vi "Test - FGV - Test Results.vi"(7 "Get/Set":T2, 8 "error in (no error)":errorcluster, 10 "Step Result":T1={"Step Name"="", "Value"=0.0, "Success ?"=TRUE, "Stop Seq ?"=FALSE, "Abort"=FALSE, "Sr.No"=0}) -> (0 "error out":errorcluster, 2 "Results":T1[](array[typedef]))   [LabVIEW 2017]
uses:
  Test - Step Result.ctl
  Controls/RT- Get Set.ctl
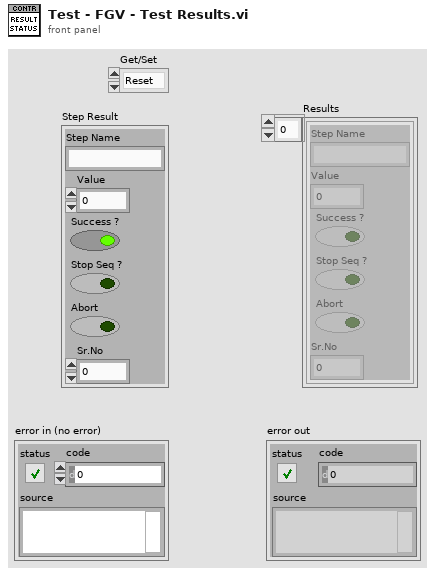
[diagram p1: front panel]
types:
  T1 = typedef "Test - Step Result.ctl" = cluster{"Step Name":string, "Value":dbl, "Success ?":bool, "Stop Seq ?":bool, "Abort":bool, "Sr.No":i32}
  T2 = typedef "RT- Get Set.ctl" = enum16{"Reset", "Get", "Set"}
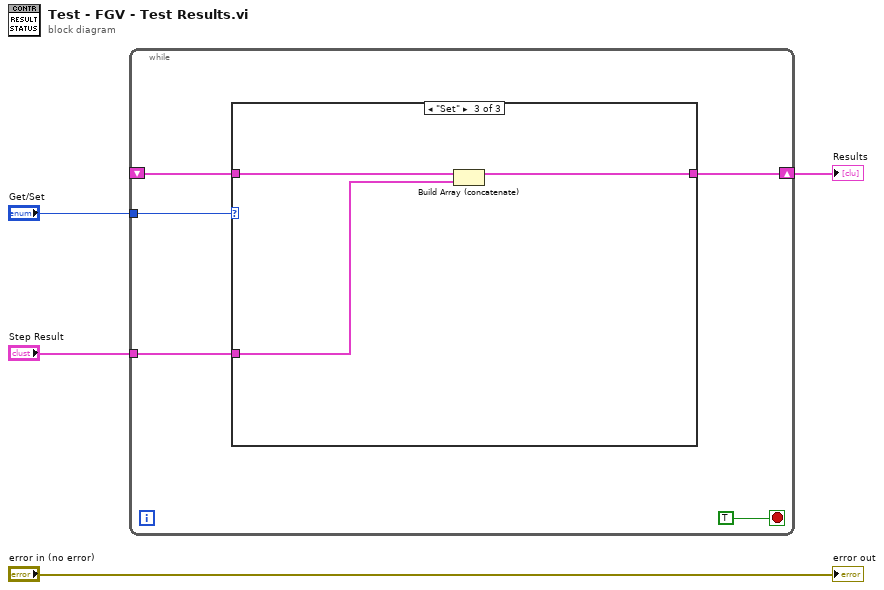
[diagram p0: block diagram]
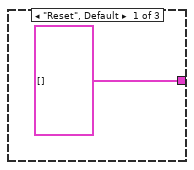
[diagram p2: hidden frame]
diagram:
  n1 = while {
    tunnel: "Get/Set" -> [w8]
    shift-right: [w7] -> w1
    shift-left: _ -> [w6]
    tunnel: "Step Result" -> [w5]
    stop <- TRUE stop-if-true
    n2 = case shown="\"Set\"" w8 {
      tunnel: [T1[] [] w11 w12] -> w7
      tunnel: w6 -> [_ w11 w14]
      tunnel: w5 -> [_ _ w13]
      frame "Reset", Default {
      }
      frame "Get" {
      }
      frame "Set" {
        n3 = Build Array (concatenate)(w14, w13) -> (w12:T1[])
      }
    }
  }
  "Results" <- w1
  "error out" <- "error in (no error)"
